vi "获取具体消息.vi"(1 "URL":string, 2 "error in (no error)":errorcluster caption="错误输入（无错误）") -> (0 "body":string, 4 "type":dbl, 5 "image_source":string, 6 "css":string[](array[string]), 7 "title":string, 8 "id":dbl, 9 "image":string, 10 "error out":errorcluster caption="错误输出", 11 "share_url":string, 12 "recommenders":string[](array[string]), 13 "ga_prefix":string, 14 "section":T1)   [LabVIEW 2012]
uses:
  <vilib>/addons/JSON API/JSON Value/JSON Value.lvclass
  <vilib>/addons/JSON API/JSON Value/Set from JSON string.vi
  <vilib>/addons/JSON API/Get Polymorphic/JSON GetSet.lvlib
  <vilib>/addons/JSON API/JSON Scalar/JSON Scalar.lvclass
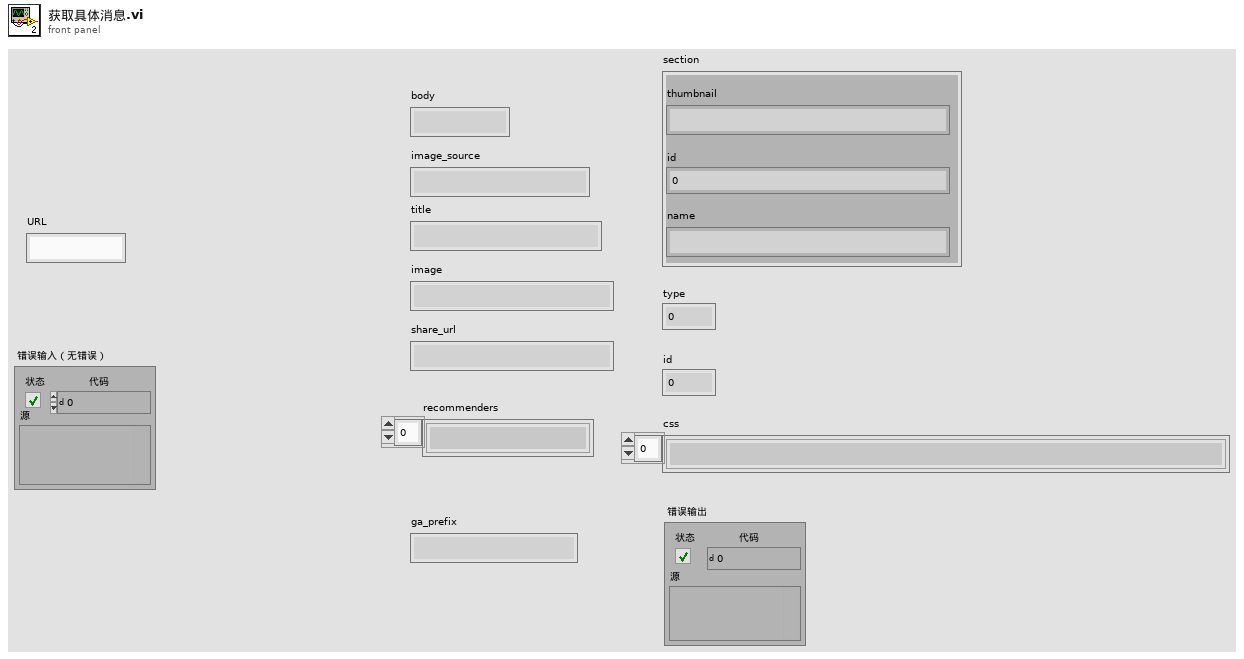
[diagram p1: front panel]
types:
  T1 = cluster{"thumbnail":string, "id":i64, "name":string}
  T2 = cluster{"LabVIEW Text":string, "Number":i32, "LabVIEW Text":string}
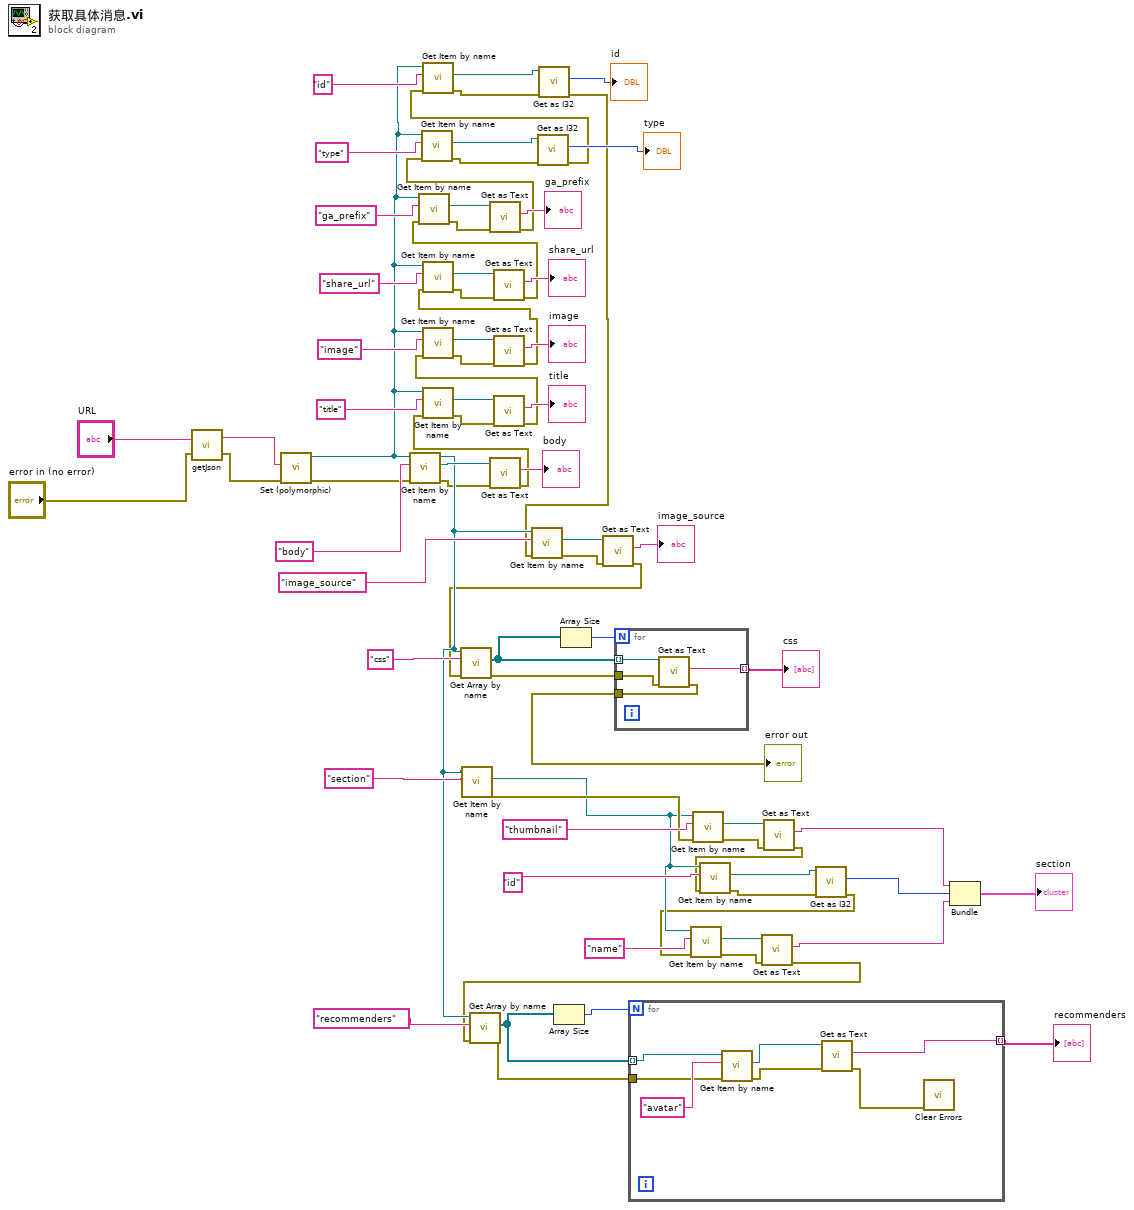
[diagram p0: block diagram]
diagram:
  n1 = call "getJson.vi"("error in (no error)"="error in (no error)", "URL"="URL") -> ("error out"=w69:errorcluster, "响应体"=w70:string)
  n2 = call-poly <vilib>:"Set (polymorphic).vi"("error in (no error)"=w69, "JSON stream"=w70) -> ("error out"=w19:errorcluster, "JSON Value out"=w47:refnum<class "JSON Value.lvclass">)  [unwired: 7 in, 1 out]
  n3 = call-dynamic "Get Item by name.vi"("error in (no error)"=w19, "name"="body", "JSON Value In"=w47) -> ("error out"=w18:errorcluster, "Value"=w75:refnum<class "JSON Value.lvclass">, "JSON Value Out"=w29:refnum<class "JSON Value.lvclass">)  [unwired: 5 in, 1 out]
  n4 = call-dynamic "Get Item by name.vi"("name"="section", "JSON Value In"=w29) -> ("error out"=w32:errorcluster, "Value"=w24:refnum<class "JSON Value.lvclass">)  [unwired: 6 in, 2 out]
  n5 = call <vilib>:"Get as Text.vi"("error in (no error)"=w18, "JSON Scalar in"=w75) -> ("error out"=w17:errorcluster, "LabVIEW Text"=→"body":string)  [unwired: 7 in, 1 out]
  n6 = call-dynamic "Get Item by name.vi"("error in (no error)"=w17, "name"="title", "JSON Value In"=w47) -> ("error out"=w16:errorcluster, "Value"=w63:refnum<class "JSON Value.lvclass">)  [unwired: 5 in, 2 out]
  n7 = call <vilib>:"Get as Text.vi"("error in (no error)"=w16, "JSON Scalar in"=w63) -> ("error out"=w15:errorcluster, "LabVIEW Text"=→"title":string)  [unwired: 7 in, 1 out]
  n8 = call-dynamic "Get Item by name.vi"("error in (no error)"=w15, "name"="image", "JSON Value In"=w47) -> ("error out"=w14:errorcluster, "Value"=w60:refnum<class "JSON Value.lvclass">)  [unwired: 5 in, 2 out]
  n9 = call <vilib>:"Get as Text.vi"("error in (no error)"=w14, "JSON Scalar in"=w60) -> ("error out"=w13:errorcluster, "LabVIEW Text"=→"image":string)  [unwired: 7 in, 1 out]
  n10 = call-dynamic "Get Item by name.vi"("error in (no error)"=w13, "name"="share_url", "JSON Value In"=w47) -> ("error out"=w12:errorcluster, "Value"=w57:refnum<class "JSON Value.lvclass">)  [unwired: 5 in, 2 out]
  n11 = call <vilib>:"Get as Text.vi"("error in (no error)"=w12, "JSON Scalar in"=w57) -> ("error out"=w11:errorcluster, "LabVIEW Text"=→"share_url":string)  [unwired: 7 in, 1 out]
  n12 = call-dynamic "Get Item by name.vi"("error in (no error)"=w11, "name"="ga_prefix", "JSON Value In"=w47) -> ("error out"=w10:errorcluster, "Value"=w54:refnum<class "JSON Value.lvclass">)  [unwired: 5 in, 2 out]
  n13 = call <vilib>:"Get as Text.vi"("error in (no error)"=w10, "JSON Scalar in"=w54) -> ("error out"=w9:errorcluster, "LabVIEW Text"=→"ga_prefix":string)  [unwired: 7 in, 1 out]
  n14 = call-dynamic "Get Item by name.vi"("error in (no error)"=w9, "name"="type", "JSON Value In"=w47) -> ("error out"=w8:errorcluster, "Value"=w50:refnum<class "JSON Value.lvclass">)  [unwired: 5 in, 2 out]
  n15 = call <vilib>:"Get as I32.vi"("error in (no error)"=w8, "JSON Scalar in"=w50) -> ("error out"=w7:errorcluster, "Number"=→"type":i32)  [unwired: 7 in, 1 out]
  n16 = call-dynamic "Get Item by name.vi"("error in (no error)"=w7, "name"="id", "JSON Value In"=w47) -> ("error out"=w6:errorcluster, "Value"=w48:refnum<class "JSON Value.lvclass">)  [unwired: 5 in, 2 out]
  n17 = call <vilib>:"Get as I32.vi"("error in (no error)"=w6, "JSON Scalar in"=w48) -> ("error out"=w5:errorcluster, "Number"=→"id":i32)  [unwired: 7 in, 1 out]
  n18 = call-dynamic "Get Item by name.vi"("error in (no error)"=w5, "name"="image_source", "JSON Value In"=w29) -> ("error out"=w65:errorcluster, "Value"=w66:refnum<class "JSON Value.lvclass">)  [unwired: 5 in, 2 out]
  n19 = call <vilib>:"Get as Text.vi"("error in (no error)"=w65, "JSON Scalar in"=w66) -> ("error out"=w4:errorcluster, "LabVIEW Text"=→"image_source":string)  [unwired: 7 in, 1 out]
  n20 = call <vilib>:"Get Array by name.vi"("error in (no error)"=w4, "name"="css", "JSON Value In"=w29) -> ("error out"=w3:errorcluster, "Array"=w71:refnum<class "JSON Value.lvclass">[])  [unwired: 5 in, 2 out]
  n21 = Array Size(array=w71) -> (size(s)=w72:i32)
  n22 = for {
    N: w72 -> [_]
    tunnel: w71 -> [w81] mode=indexing
    tunnel: [w80] -> w33 mode=indexing
    tunnel: w3 -> [w79]
    tunnel: [w78] -> w1
    n23 = call <vilib>:"Get as Text.vi"("error in (no error)"=w79, "JSON Scalar in"=w81) -> ("error out"=w78:errorcluster, "LabVIEW Text"=w80:string)  [unwired: 7 in, 1 out]
  }
  "css" <- w33
  "error out" <- w1
  n24 = call-dynamic "Get Item by name.vi"("error in (no error)"=w32, "name"="thumbnail", "JSON Value In"=w24) -> ("error out"=w44:errorcluster, "Value"=w45:refnum<class "JSON Value.lvclass">)  [unwired: 5 in, 2 out]
  n25 = call <vilib>:"Get as Text.vi"("error in (no error)"=w44, "JSON Scalar in"=w45) -> ("error out"=w20:errorcluster, "LabVIEW Text"=w37:string)  [unwired: 7 in, 1 out]
  n26 = call-dynamic "Get Item by name.vi"("error in (no error)"=w20, "name"="id", "JSON Value In"=w24) -> ("error out"=w23:errorcluster, "Value"=w41:refnum<class "JSON Value.lvclass">)  [unwired: 5 in, 2 out]
  n27 = call <vilib>:"Get as I32.vi"("error in (no error)"=w23, "JSON Scalar in"=w41) -> ("error out"=w22:errorcluster, "Number"=w36:i32)  [unwired: 7 in, 1 out]
  n28 = call-dynamic "Get Item by name.vi"("error in (no error)"=w22, "name"="name", "JSON Value In"=w24) -> ("error out"=w39:errorcluster, "Value"=w40:refnum<class "JSON Value.lvclass">)  [unwired: 5 in, 2 out]
  n29 = call <vilib>:"Get as Text.vi"("error in (no error)"=w39, "JSON Scalar in"=w40) -> ("error out"=w21:errorcluster, "LabVIEW Text"=w35:string)  [unwired: 7 in, 1 out]
  n30 = call <vilib>:"Get Array by name.vi"("error in (no error)"=w21, "name"="recommenders", "JSON Value In"=w29) -> ("error out"=w2:errorcluster, "Array"=w26:refnum<class "JSON Value.lvclass">[])  [unwired: 5 in, 2 out]
  n31 = Array Size(array=w26) -> (size(s)=w27:i32)
  n32 = for {
    N: w27 -> [_]
    tunnel: [w88] -> w25 mode=indexing
    tunnel: w26 -> [w87] mode=indexing
    tunnel: w2 -> [w82]
    n33 = call-dynamic "Get Item by name.vi"("error in (no error)"=w82, "name"="avatar", "JSON Value In"=w87) -> ("error out"=w84:errorcluster, "Value"=w85:refnum<class "JSON Value.lvclass">)  [unwired: 5 in, 2 out]
    n34 = call <vilib>:"Get as Text.vi"("error in (no error)"=w84, "JSON Scalar in"=w85) -> ("error out"=w83:errorcluster, "LabVIEW Text"=w88:string)  [unwired: 7 in, 1 out]
    n35 = call <vilib>:"Clear Errors.vi"("error in (no error)"=w83) -> ()  [unwired: 6 in, 1 out]
  }
  "recommenders" <- w25
  n36 = Bundle("LabVIEW Text"=w37, "Number"=w36, "LabVIEW Text"=w35) -> (→"section":T2)  [unwired: 1 in]
